vi "_Update Display Property 2.vi"(7 "Spectrum in":i32[](array[numeric])) -> ()   [LabVIEW 2012]
uses:
  Configuration/_Global Configuration.vi
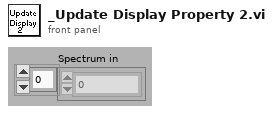
[diagram p1: front panel]
types:
  T1 = typedef "_Lens Property.ctl" = cluster{"Scan Type":u8, "Scans":i32, "Time 1":dbl, "Time 2":dbl, "Value 1":dbl, "Value 2":dbl, "Step Size":dbl}
  T2 = typedef "_Mass Range Property.ctl" = cluster{"Start":dbl, "Stop":dbl, "Step Size":dbl, "Steps":i32, "Dwell":dbl, "Parameters":T3[], "Res":T4}
  T3 = typedef "_Mass Range Parameters.ctl" = cluster{"Name":string, "Ch#":u8, "StartV":dbl, "StopV":dbl, "StepV":dbl, "Index":u8}
  T4 = typedef "_RT Res Type.ctl" = u16
  T5 = typedef "_Run Mode.ctl" = enum16{"MRM (Q1/Q2)", "Q1 Scan", "Q1 SRM", "Q2 Scan", "Q2 SRM", "Product Scan", "Precursor Scan", "Neutral Loss", "Neutral Gain"}
  T6 = cluster{"Lenses":T1[], "Mass Ranges":T2[], "Acquire":bool, "MCA":bool, "Q1DC EN":bool, "Q1 POL":bool, "Q3 POL":bool, "Q1 RF  EN":bool, "Averaging":bool, "Log Scale":bool, "CPS":bool, "Unit":bool, "Data Path":path, "Run Mode":T5, "Fixed Mass (amu)":dbl, "Q3DC EN":bool, "Q3 RF  EN":bool, "Negative":bool}
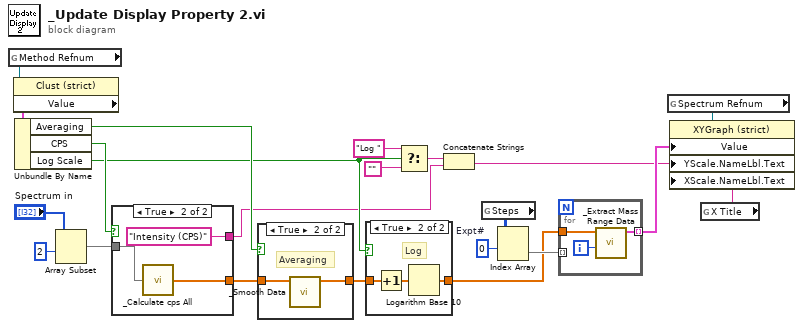
[diagram p0: block diagram]
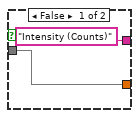
[diagram p4: hidden frame]
diagram:
  w7 = 0  # Expt#
  n1 = global read "_Global Configuration.vi" "Method Refnum"() -> (w22:refnum<vi>)
  n2 = property class="Clust (strict)"(reference=w22) -> ("Value"=w21:T6)  [unwired: 1 in, 2 out]
  n3 = Unbundle By Name(w21) -> ("Averaging"=w20:bool, "CPS"=w19:bool, "Log Scale"=w13:bool)
  n4 = Array Subset(array="Spectrum in", index=2) -> (w9:i32[])  [unwired: 1 in]
  n5 = case shown="True" w19 {
    tunnel: [w23 w25] -> w18
    tunnel: ["Intensity (Counts)" "Intensity (CPS)"] -> w12
    tunnel: w9 -> [w23 w26]
    frame False {
    }
    frame True {
      n6 = call "_Calculate cps All.vi"("Raw Counts"=w26) -> ("Data in cps"=w25:dbl[])
    }
  }
  n7 = case shown="True" w20 {
    tunnel: w18 -> [w28 w30]
    tunnel: [w28 w29] -> w17
    frame False {
    }
    frame True {
      # "Averaging"
      n8 = call "_Smooth Data.vi"("Data In"=w30) -> ("Data Out"=w29:dbl[])  [unwired: 6 out]
    }
  }
  n9 = case shown="True" w13 {
    tunnel: w17 -> [w31 w34]
    tunnel: [w31 w33] -> w5
    frame False {
    }
    frame True {
      # "Log"
      n10 = Increment(x=w34) -> (x+1=w32:dbl[])
      n11 = Logarithm Base 10(1:w32) -> (0:w33:dbl[])
    }
  }
  n12 = Select(t="Log ", s=w13, f="") -> (s? t:f=w16:string)
  n13 = Concatenate Strings(w16, w12) -> (w1:string)
  n14 = global read "_Global Configuration.vi" "Steps"() -> (w8:i32[][])
  n15 = Index Array(array=w8, index (row)=w7) -> (element=w6:i32[])  [unwired: 1 in]
  n16 = for {
    tunnel: w6 -> [_] mode=indexing
    tunnel: w5 -> [w36]
    tunnel: [w35] -> w2 mode=indexing
    i -> [w37]
    n17 = call "_Extract Mass Range Data.vi"("MR# (0)"=w37, "Spectrum"=w36) -> ("MR Data"=w35:cluster{dbl[], dbl[]})  [unwired: 1 in, 4 out]
  }
  n18 = global read "_Global Configuration.vi" "Spectrum Refnum"() -> (w4:refnum<vi>)
  n19 = global read "_Global Configuration.vi" "X Title"() -> (w3:string)
  n20 = property class="XYGraph (strict)"(reference=w4, "Value"=w2, "YScale.NameLbl.Text"=w1, "XScale.NameLbl.Text"=w3) -> ()  [unwired: 1 in, 2 out]
